vi "Hall_Screen.vi"(0 "Model":string, 1 "Write":refnum<k21>, 2 "Read":refnum<k21>, 3 "Numeric":dbl, 4 "Numeric Request":u32) -> (5 "Read out":refnum<k21>, 6 "Write out":refnum<k21>)   [LabVIEW 2023]
panel:
  in  "OK":bool
  out "String":string
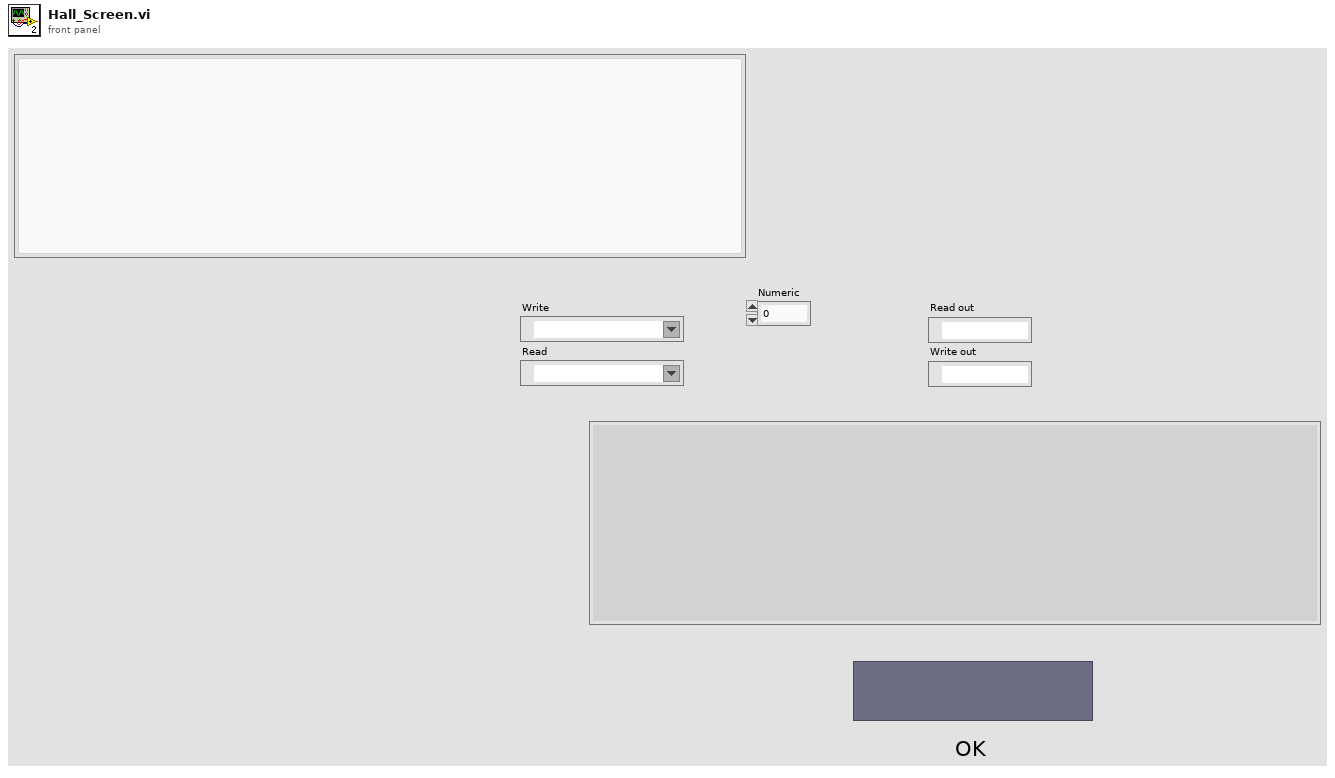
[diagram p1: front panel]
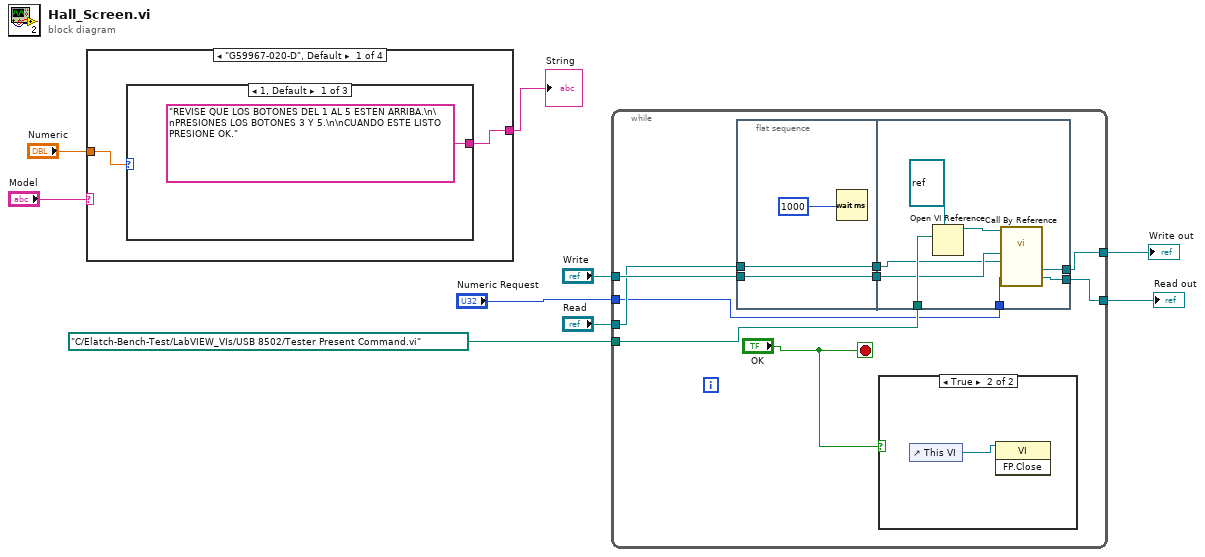
[diagram p0: block diagram]
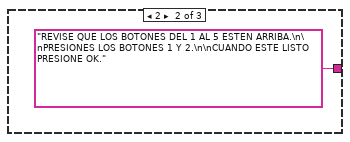
[diagram p3: hidden frame]
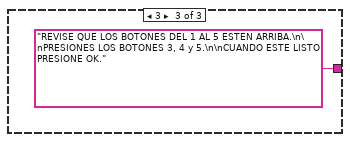
[diagram p4: hidden frame]
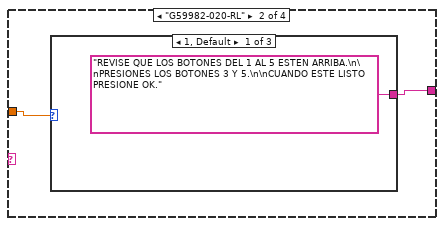
[diagram p5: hidden frame]
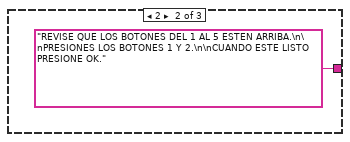
[diagram p6: hidden frame]
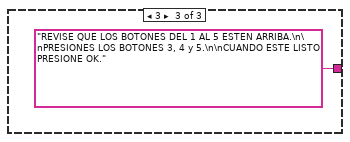
[diagram p7: hidden frame]
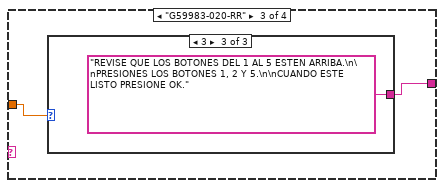
[diagram p8: hidden frame]
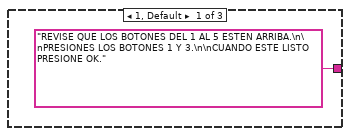
[diagram p9: hidden frame]
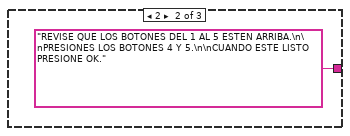
[diagram p10: hidden frame]
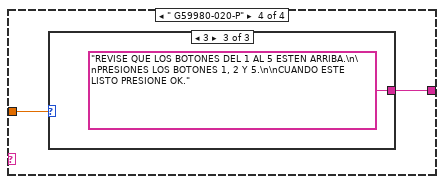
[diagram p11: hidden frame]
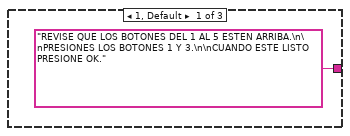
[diagram p12: hidden frame]
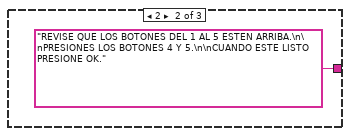
[diagram p13: hidden frame]
diagram:
  n1 = case shown="\"G59967-020-D\", Default" "Model" {
    tunnel: "Numeric" -> [w11 w16 w21 w26]
    tunnel: [w10 w15 w20 w25] -> w6
    frame "G59967-020-D", Default {
      n2 = case shown="1, Default" w11 {
        tunnel: ["REVISE QUE LOS BOTONES DEL 1 AL 5 ESTEN ARRIBA.\n\nPRESIONES LOS BOTONES 3 Y 5.\n\nCUANDO ESTE LISTO PRESIONE OK." ("Message") "REVISE QUE LOS BOTONES DEL 1 AL 5 ESTEN ARRIBA.\n\nPRESIONES LOS BOTONES 1 Y 2.\n\nCUANDO ESTE LISTO PRESIONE OK." ("Message") "REVISE QUE LOS BOTONES DEL 1 AL 5 ESTEN ARRIBA.\n\nPRESIONES LOS BOTONES 3, 4 y 5.\n\nCUANDO ESTE LISTO PRESIONE OK." ("Message")] -> w10
        frame 1, Default {
        }
        frame 2 {
        }
        frame 3 {
        }
      }
    }
    frame "G59982-020-RL" {
      n3 = case shown="1, Default" w16 {
        tunnel: ["REVISE QUE LOS BOTONES DEL 1 AL 5 ESTEN ARRIBA.\n\nPRESIONES LOS BOTONES 3 Y 5.\n\nCUANDO ESTE LISTO PRESIONE OK." ("Message") "REVISE QUE LOS BOTONES DEL 1 AL 5 ESTEN ARRIBA.\n\nPRESIONES LOS BOTONES 1 Y 2.\n\nCUANDO ESTE LISTO PRESIONE OK." ("Message") "REVISE QUE LOS BOTONES DEL 1 AL 5 ESTEN ARRIBA.\n\nPRESIONES LOS BOTONES 3, 4 y 5.\n\nCUANDO ESTE LISTO PRESIONE OK." ("Message")] -> w15
        frame 1, Default {
        }
        frame 2 {
        }
        frame 3 {
        }
      }
    }
    frame "G59983-020-RR" {
      n4 = case shown="3" w21 {
        tunnel: ["REVISE QUE LOS BOTONES DEL 1 AL 5 ESTEN ARRIBA.\n\nPRESIONES LOS BOTONES 1 Y 3.\n\nCUANDO ESTE LISTO PRESIONE OK." ("Message") "REVISE QUE LOS BOTONES DEL 1 AL 5 ESTEN ARRIBA.\n\nPRESIONES LOS BOTONES 4 Y 5.\n\nCUANDO ESTE LISTO PRESIONE OK." ("Message") "REVISE QUE LOS BOTONES DEL 1 AL 5 ESTEN ARRIBA.\n\nPRESIONES LOS BOTONES 1, 2 Y 5.\n\nCUANDO ESTE LISTO PRESIONE OK." ("Message")] -> w20
        frame 1, Default {
        }
        frame 2 {
        }
        frame 3 {
        }
      }
    }
    frame " G59980-020-P" {
      n5 = case shown="3" w26 {
        tunnel: ["REVISE QUE LOS BOTONES DEL 1 AL 5 ESTEN ARRIBA.\n\nPRESIONES LOS BOTONES 1 Y 3.\n\nCUANDO ESTE LISTO PRESIONE OK." ("Message") "REVISE QUE LOS BOTONES DEL 1 AL 5 ESTEN ARRIBA.\n\nPRESIONES LOS BOTONES 4 Y 5.\n\nCUANDO ESTE LISTO PRESIONE OK." ("Message") "REVISE QUE LOS BOTONES DEL 1 AL 5 ESTEN ARRIBA.\n\nPRESIONES LOS BOTONES 1, 2 Y 5.\n\nCUANDO ESTE LISTO PRESIONE OK." ("Message")] -> w25
        frame 1, Default {
        }
        frame 2 {
        }
        frame 3 {
        }
      }
    }
  }
  "String" <- w6
  n6 = while {
    tunnel: "Read" -> [w37]
    tunnel: "Write" -> [w38]
    tunnel: path "C:/Elatch-Bench-Test/LabVIEW_VIs/USB 8502/Tester Present Command.vi" ("vi path") -> [w34]
    tunnel: [w32] -> w3
    tunnel: [w31] -> w2
    tunnel: "Numeric Request" -> [w30]
    stop <- "OK" stop-if-true
    n7 = flat-sequence {
      tunnel: w37 -> [w40]
      tunnel: w38 -> [w41]
      tunnel: [w41] -> w36
      tunnel: [w40] -> w35
      tunnel: w36 -> [w46]
      tunnel: w35 -> [w45]
      tunnel: w34 -> [w49]
      tunnel: [w44] -> w32
      tunnel: [w43] -> w31
      tunnel: w30 -> [w42]
      frame #0 {
        n8 = Wait (ms)(milliseconds to wait=u32 1000) -> ()  [unwired: 1 out]
      }
      frame #1 {
        n9 = Open VI Reference(type specifier VI Refnum (for type only)=refnum<vi> refnum, vi path=w49) -> (vi reference=w47:refnum<vi>)  [unwired: 4 in, 1 out]
        n10 = call-by-ref "?"(reference=w47, "Numeric Request"=w42, "Read"=w45, "Write"=w46) -> ("Read out"=w43:refnum<k21>, "Write out"=w44:refnum<k21>)  [unwired: 3 in, 4 out]
      }
    }
    n11 = case shown="True" "OK" {
      frame False {
      }
      frame True {
        n12 = control-ref of="This VI"() -> (w50:refnum<vi>)
        n13 = invoke class="VI" method="FP.Close"(reference=w50) -> ()  [unwired: 2 in, 3 out]
      }
    }
  }
  "Write out" <- w3
  "Read out" <- w2
